vi "Close MeasurementLink Session.vi"(8 "error in":errorcluster, 9 "initialize and close session behavior":T1, 10 "session in":variant, 11 "session factory in":refnum<class "ISession Factory.lvclass">) -> (0 "error out":errorcluster)   [LabVIEW 2021, in "NI Session Management Instrument.lvlib" / "ISession Factory.lvclass"]
doc: "Closes the local session. If the session represents a remote session, <b>initialize and close session behavior</b> determines whether closing the local session closes the server session or detaches from the server session."
uses:
  ISession Factory.lvclass
  Initialize and Close Session Behavior.ctl
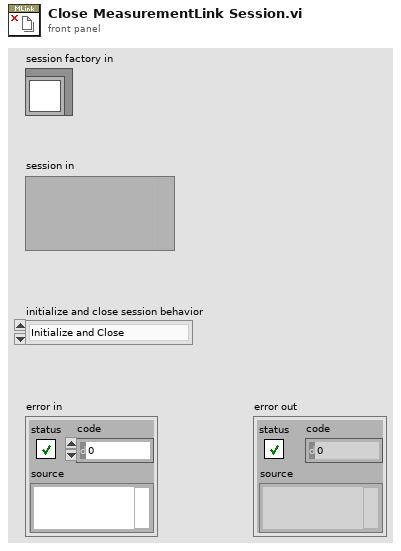
[diagram p1: front panel]
types:
  T1 = typedef "NI Session Management Instrument.lvlib/ISession Factory.lvclass/Initialize and Close Session Behavior.ctl" = enum16{"Initialize and Close", "Attach and Detach", "Initialize and Detach", "Attach and Close"}
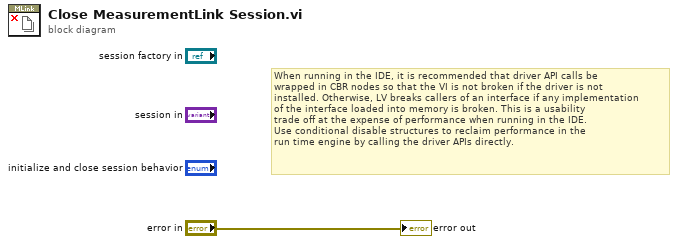
[diagram p0: block diagram]
diagram:
  # "When running in the IDE, it is recommended that driver API calls be \nwrapped in CBR nodes so that the VI is not broken if the driver is not \ninstalled. Otherwise, LV breaks callers of an interface if any implementation\nof the interface loaded into memory is broken. This is a usability\ntrade off at the expense of performance when running in the IDE.\nUse conditional disable structures to reclaim performance in the \nrun time engine by calling the driver APIs directly."
  "error out" <- "error in"
